vi "Msg.vi"(7 "Actor in":refnum<class "Actor.lvclass">, 11 "Last Ack Msg in":refnum<class "Last Ack Msg.lvclass">) -> (5 "Actor out":refnum<class "Actor.lvclass">)   [LabVIEW 2020, in "jettl.lvlib" / "Last Ack Msg.lvlib" / "Last Ack Msg.lvclass"]
uses:
  Last Ack Msg.lvclass
  Actor/Actor/Actor.lvclass
  Last Ack/Last Ack.lvclass
  Last Ack Msg.lvclass/Last Ack Msg.ctl
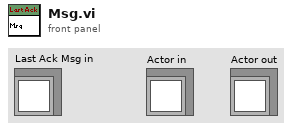
[diagram p1: front panel]
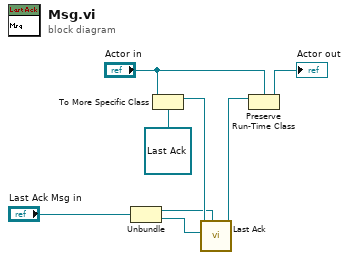
[diagram p0: block diagram]
diagram:
  n1 = Unbundle "Unbundle"("Last Ack Msg in") -> (w1:refnum<class "Sender.lvclass">, w2:refnum<class "Actor.lvclass">)
  n2 = To More Specific Class(target class=refnum<class "Last Ack.lvclass"> refnum ("jettl.lvlib:jettl Msg Last Ack Creator Queue.lvlib:jettl Msg Last Ack Creator Queue.lvclass"), reference="Actor in") -> (specific class reference=w4:refnum<class "Last Ack.lvclass">)  [unwired: 1 in, 1 out]
  n3 = call-dynamic "Last Ack.vi"("Sender"=w1, "Actor"=w2, "Last Ack in"=w4) -> ("Last Ack out"=w3:refnum<class "Last Ack.lvclass">)  [unwired: 8 in]
  n4 = Preserve Run-Time Class(object in=w3, 2:"Actor in") -> (object out=→"Actor out":refnum<class "Actor.lvclass">)  [unwired: 1 in, 1 out]
